vi "Initalize Data.vi"() -> (4 "Queue out":refnum<queue>, 6 "Names":string[](array[string]), 8 "VI or executable installation directory":path, 10 "Display":string[][](array[string]), 15 "error out":errorcluster)   [LabVIEW 2015]
panel:
  out "Display Path":path
  out "List Path":path
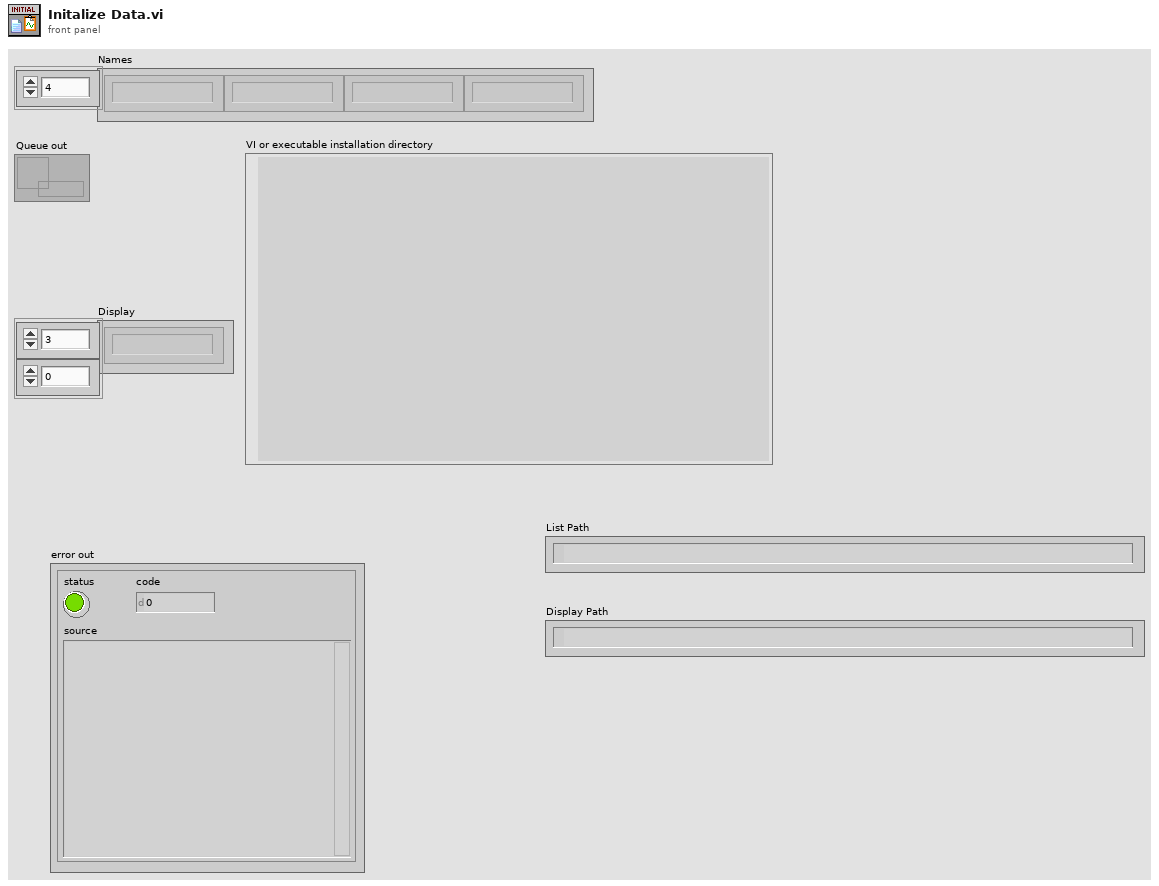
[diagram p1: front panel]
types:
  T1 = enum16{"open", "replace", "create", "open or create", "replace or create", "replace or create with confirmation"}
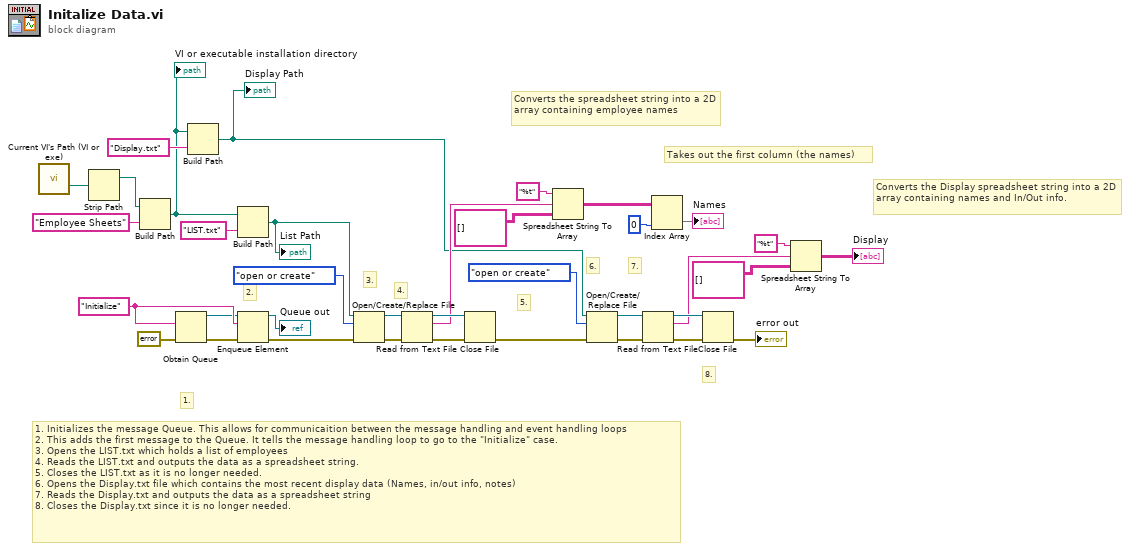
[diagram p0: block diagram]
diagram:
  w13 = "Initialize"
  # "Converts the Display spreadsheet string into a 2D array containing names and In/Out info."
  # "Takes out the first column (the names)"
  # "Converts the spreadsheet string into a 2D array containing employee names"
  # "8."
  # "7."
  # "6."
  # "5."
  # "1. Initializes the message Queue. This allows for communicaition between the message handling and event handling loops\n2. This adds the first message to the Queue. It tells the message handling loop to go to the \"Initialize\" case.\n3. Opens the LIST.txt which holds a list of employees\n4. Reads the LIST.txt and outputs the data as a spreadsheet string.\n5. Closes the LIST.txt as it is no longer needed.\n6. Opens the Display.txt file which contains the most recent display data (Names, in/out info, notes)\n7. Reads the Display.txt and outputs the data as a spreadsheet string\n8. Closes the Display.txt since it is no longer needed."
  # "4."
  # "3."
  # "2."
  # "1."
  n1 = call "Current VI's Path (VI or exe).vi"() -> ("VI or executable installation directory"=w8:path)  [unwired: 14 in, 1 out]
  n2 = Strip Path(path=w8) -> (stripped path=w3:path)  [unwired: 1 out]
  n3 = Build Path(base path=w3, name or relative path="Employee Sheets") -> (appended path=w1:path)
  "VI or executable installation directory" <- w1
  n4 = Obtain Queue(element data type=w13, error in (no error)=errorcluster {"status"=FALSE, "code"=0, "source"=""}) -> (queue out=w11:refnum<queue>, error out=w10:errorcluster)  [unwired: 3 in, 1 out]
  n5 = Build Path(base path=w1, name or relative path="Display.txt") -> (appended path=w4:path)
  "Display Path" <- w4
  n6 = Build Path(base path=w1, name or relative path="LIST.txt") -> (appended path=w6:path)
  "List Path" <- w6
  n7 = Enqueue Element(queue=w11, element=w13, error in (no error)=w10) -> (queue out=→"Queue out":refnum<queue>, error out=w21:errorcluster)  [unwired: 1 in, 1 out]
  n8 = Open/Create/Replace File(file path (use dialog)=w6, error in=w21, operation (0:open)=T1."open or create") -> (refnum out=w15:refnum<file>, error out=w20:errorcluster)  [unwired: 3 in, 1 out]
  n9 = Read from Text File(file (use dialog)=w15, error in=w20) -> (refnum out=w18:refnum<file>, text=w17:string, error out=w36:errorcluster)  [unwired: 2 in, 1 out]
  n10 = Close File(refnum=w18, error in=w36) -> (error out=w35:errorcluster)  [unwired: 1 out]
  n11 = Spreadsheet String To Array(format string="%t", spreadsheet string=w17, array type (2D Dbl)=string[][] []) -> (array=w23:string[][])  [unwired: 1 in]
  n12 = Open/Create/Replace File(file path (use dialog)=w4, error in=w35, operation (0:open)=T1."open or create") -> (refnum out=w28:refnum<file>, error out=w27:errorcluster)  [unwired: 3 in, 1 out]
  n13 = Read from Text File(file (use dialog)=w28, error in=w27) -> (refnum out=w32:refnum<file>, text=w29:string, error out=w31:errorcluster)  [unwired: 2 in, 1 out]
  n14 = Index Array(array=w23, index (col)=0 ("disabled index (col)")) -> (element=→"Names":string[])  [unwired: 1 in]
  n15 = Close File(refnum=w32, error in=w31) -> (error out=→"error out":errorcluster)  [unwired: 1 out]
  n16 = Spreadsheet String To Array(format string="%t", spreadsheet string=w29, array type (2D Dbl)=string[][] []) -> (array=→"Display":string[][])  [unwired: 1 in]
